vi "Error if not a Host Key Database.vi"(8 "error in (no error)":errorcluster, 11 "host key database":T1) -> (0 "error out":errorcluster, 3 "host key database out":T1)   [LabVIEW 2017, in "libssh2.lvlib"]
doc: "Reports an error if <B>known host collection</B> is not a known host collection."
uses:
  libssh2.lvlib
  Host Key Database Refnum.ctl
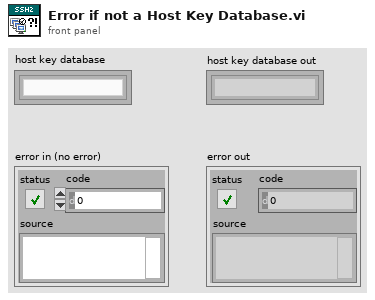
[diagram p1: front panel]
types:
  T1 = typedef "libssh2.lvlib/Host Key Database Refnum.ctl" = refnum<k1>
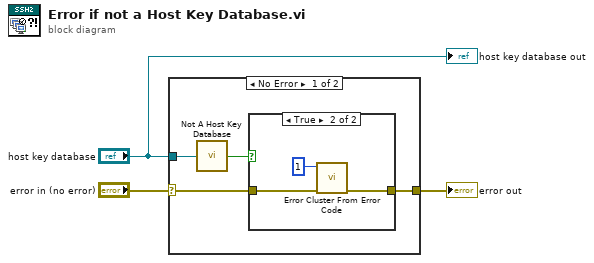
[diagram p0: block diagram]
diagram:
  n1 = case shown="No Error" "error in (no error)" {
    selector: "error in (no error)" -> [w4 w12]
    tunnel: [w7 w12] -> w3
    tunnel: "host key database" -> [w5 _]
    frame No Error {
      n2 = call "Not A Host Key Database.vi"("host key database"=w5) -> ("Not a Host Key Database?"=w6:bool)
      n3 = case shown="True" w6 {
        tunnel: w4 -> [w8 w10]
        tunnel: [w8 w9] -> w7
        frame False {
        }
        frame True {
          n4 = call <vilib>:"Error Cluster From Error Code.vi"("error in (no error)"=w10, "error code (0)"=1) -> ("error out"=w9:errorcluster)  [unwired: 7 in]
        }
      }
    }
    frame Error {
    }
  }
  "error out" <- w3
  "host key database out" <- "host key database"
